vi "Launch Image Averaging.vi"(8 "error in (no error)":errorcluster, 11 "Controller in":refnum<class "Controller.lvclass">) -> (0 "error out":errorcluster, 3 "Controller out":refnum<class "Controller.lvclass">)   [LabVIEW 2022 SP3, in "Controller.lvlib" / "Controller.lvclass"]
uses:
  Controller.lvclass
  ImageHandler/ImageHandler Messages/DeInit Msg/DeInit Msg.lvclass
  <vilib>/ActorFramework/Actor/Actor.lvclass
  ImageHandler/Image Averaging/Image Averaging.lvclass
  UserInterface/UserInterface Messages/Log Data Msg/Log Data Msg.lvclass
  C:/Program Files/National Instruments/LabVIEW 2022/vi.lib/ActorFramework/Actor/Actor.lvclass
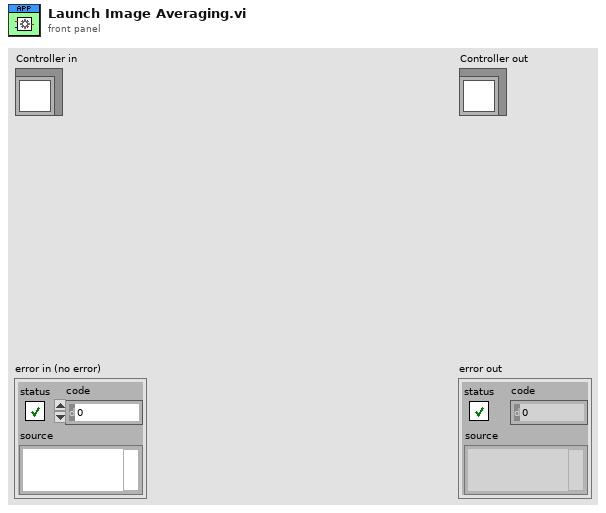
[diagram p1: front panel]
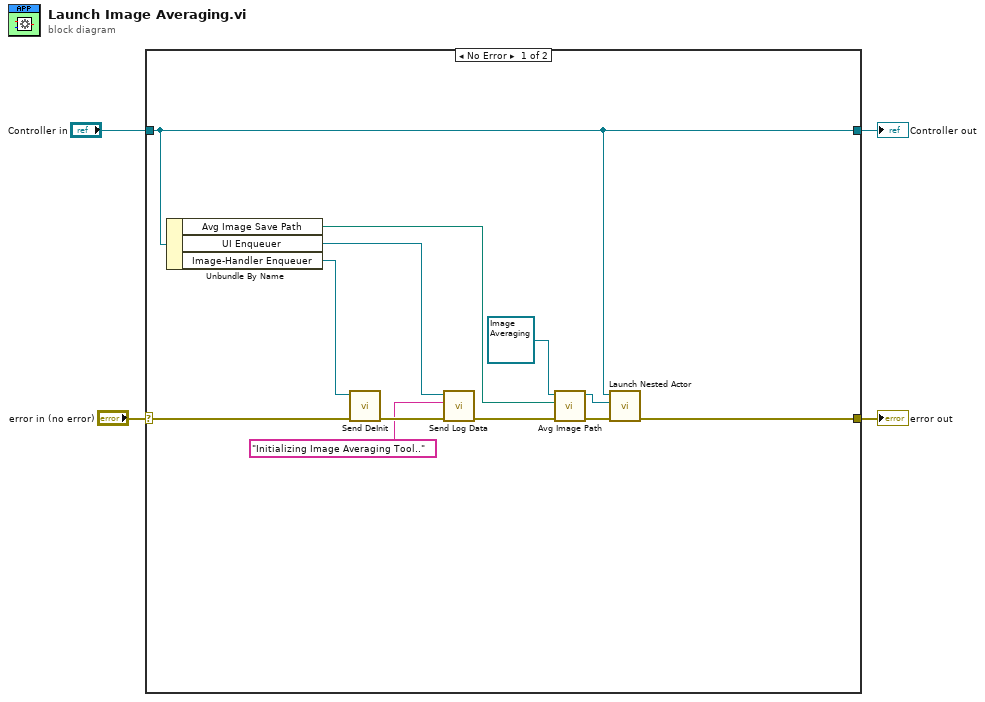
[diagram p0: block diagram]
diagram:
  n1 = case shown="No Error" "error in (no error)" {
    selector: "error in (no error)" -> [w14 w18]
    tunnel: "Controller in" -> [w12 w17]
    tunnel: [w12 w17] -> w3
    tunnel: [w13 w18] -> w2
    frame No Error {
      n2 = Unbundle By Name(w12) -> ("Avg Image Save Path"=w5:path, "UI Enqueuer"=w10:refnum<class "Message Enqueuer.lvclass">, "Image-Handler Enqueuer"=w15:refnum<class "Message Enqueuer.lvclass">)
      n3 = call "Send DeInit.vi"("error in (no error)"=w14, "Message Enqueuer"=w15) -> ("error out"=w16:errorcluster)  [unwired: 8 in, 1 out]
      n4 = call "Send Log Data.vi"("error in (no error)"=w16, "Message"="Initializing Image Averaging Tool..", "Message Enqueuer"=w10) -> ("error out"=w11:errorcluster)  [unwired: 7 in, 1 out]
      n5 = call-dynamic "Avg Image Path.vi"("error in (no error)"=w11, "Avg ImagePath"=w5, "Image Averaging in"=refnum<class "Image Averaging.lvclass"> refnum ("Image Averaging.lvlib:Image Averaging.lvclass")) -> ("error out"=w8:errorcluster, "Image Averaging out"=w6:refnum<class "Image Averaging.lvclass">)  [unwired: 7 in]
      n6 = call <vilib>:"Launch Nested Actor.vi"("error in (no error)"=w8, "Nested Actor"=w6, "Caller Actor in"=w12) -> ("error out"=w13:errorcluster)  [unwired: 6 in, 2 out]
    }
    frame Error {
    }
  }
  "error out" <- w2
  "Controller out" <- w3
